vi "Draw Rotating Dial.vi"(7 "attitude (rad)":T1, 9 "draw options":T2={"Text Color"=16777238, "Wing Color"=16751616, "Dial Outline Color"=13816530, "Sky Color"=3381759, "Ground Color"=8213043, "Horizon Line Color"=16777225, "Outline Color"=0, "Dial Background Color"=5987163, "Draw Wings"=TRUE, "Draw Text"=TRUE, "Font Name"="Helvetica", "Angle units"=enum."Radians"}, 10 "draw area state":T4={"center"={"x"=0, "y"=0}, "Thick Pen"={"Width"=0, "Style"=enum."Solid"}, "Medium Pen"={"Width"=0, "Style"=enum."Solid"}, "DrawAreaSize"={"Width"=8, "Height"=0}, "pixels per unit"=0.0, "units per radian"=0.0}, 11 "picture in":picture) -> (3 "picture out":picture)   [LabVIEW 2017, in "NI_Robotics_Attitude Picture.lvlib"]
uses:
  <vilib>/robotics/Controls/Attitude Indicator/Attitude Picture/NI_Robotics_Attitude Picture.lvlib
  <vilib>/robotics/Controls/Attitude Indicator/Attitude Picture/Draw Area State.ctl
  <vilib>/Utility/miscctls.llb/LVBoundsTypeDef.ctl
  <vilib>/robotics/Controls/Attitude Indicator/Attitude Picture/Draw Options.ctl
  <vilib>/robotics/Controls/Utilities/Angle Units.ctl
  <vilib>/robotics/Controls/Attitude Indicator/Attitude Picture/Attitude.ctl
  <vilib>/robotics/Controls/Attitude Indicator/Attitude Picture/XY to Rotated Pixel Points.vi
  <vilib>/Analysis/coordinate.llb/2D Cartesian Coordinate Rotation.vi
  <vilib>/Analysis/coordinate.llb/2D Cartesian Coordinate Rotation (Array).vi
  <vilib>/picture/picture.llb/Draw Multiple Lines.vi
  <vilib>/Utility/AngleManip/Degrees to Radians.vi
  <vilib>/Utility/AngleManip/Degrees to Radians (Scalar DBL).vi
  <vilib>/Utility/AngleManip/Degrees to Radians (Array DBL).vi
  <vilib>/robotics/Controls/Utilities/NI_Robotics_Control Utilities.lvlib
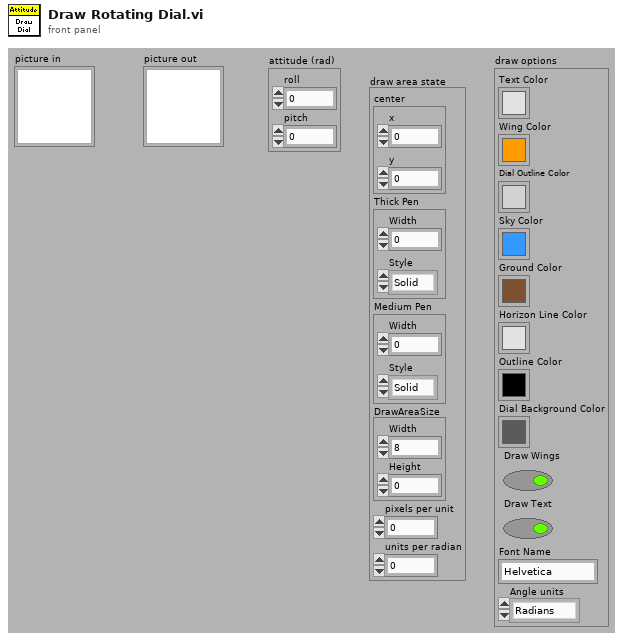
[diagram p1: front panel]
types:
  T1 = typedef "NI_Robotics_Attitude Picture.lvlib/Attitude.ctl" = cluster{"roll":dbl, "pitch":dbl}
  T2 = typedef "NI_Robotics_Attitude Picture.lvlib/Draw Options.ctl" = cluster{"Text Color":u32, "Wing Color":u32, "Dial Outline Color":u32, "Sky Color":u32, "Ground Color":u32, "Horizon Line Color":u32, "Outline Color":u32, "Dial Background Color":u32, "Draw Wings":bool, "Draw Text":bool, "Font Name":string, "Angle units":T3}
  T3 = typedef "NI_Robotics_Control Utilities.lvlib/Angle Units.ctl" = enum16{"Radians", "Degrees"}
  T4 = typedef "NI_Robotics_Attitude Picture.lvlib/Draw Area State.ctl" = cluster{"center":cluster{"x":i16, "y":i16}, "Thick Pen":cluster{"Width":u16, "Style":enum32{"Solid", "Dash", "Dot", "DashDot", "DashDotDot"}}, "Medium Pen":cluster{"Width":u16, "Style":enum32{"Solid", "Dash", "Dot", "DashDot", "DashDotDot"}}, "DrawAreaSize":T5, "pixels per unit":dbl, "units per radian":dbl}
  T5 = typedef "LVBoundsTypeDef.ctl" = cluster{"Width":u32, "Height":u32}
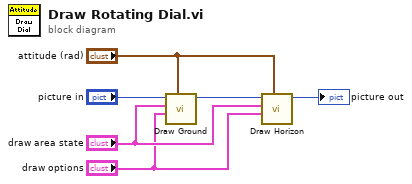
[diagram p0: block diagram]
diagram:
  n1 = call <vilib>:"Draw Ground.vi"("attitude (rad)"="attitude (rad)", "draw options"="draw options", "draw area state"="draw area state", "picture in"="picture in") -> ("picture out"=w5:picture)  [unwired: 7 in]
  n2 = call <vilib>:"Draw Horizon.vi"("attitude (rad)"="attitude (rad)", "draw options"="draw options", "draw area state"="draw area state", "picture in"=w5) -> ("picture out"=→"picture out":picture)  [unwired: 7 in]
